vi "FPGA_PPG_stop.vi"(0 "resource_in":refnum<visa-resource-name>, 5 "error in (no error)":errorcluster) -> (14 "resource_out":refnum<visa-resource-name>, 16 "stop_addr":u32, 19 "error out":errorcluster)   [LabVIEW 2014, in "NI-FPGA_PPG_Driver.lvlib"]
doc: "Stops the FPGA and returns the last executed command specified by address.\n\nContact: Falk Ziegler, eMail: ziegler@physik.uni-greifswald.de"
uses:
  NI-FPGA_PPG_Driver.lvlib
  <vilib>/Utility/error.llb/Error Cluster From Error Code.vi
  <vilib>/rvi/errors/niLvFpgaAdjustHostInterfaceError.vi
  <vilib>/rvi/interface/nirviReadWriteControl/nirviReadWriteControl.xnode
  FPGA_PPG_vi_ref.ctl
  FPGA Bitfiles/TiTaProj_COF_PPG_d3vptxinz-s.lvbitx
  NiFpgaLv.dll
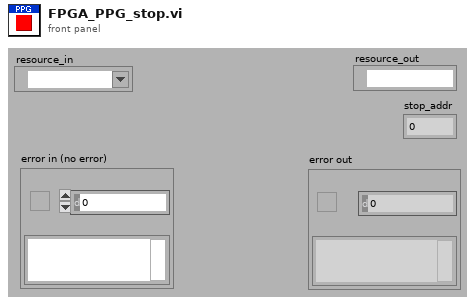
[diagram p1: front panel]
types:
  T1 = typedef "NI-FPGA_PPG_Driver.lvlib/FPGA_PPG_vi_ref.ctl" = refnum<k20>
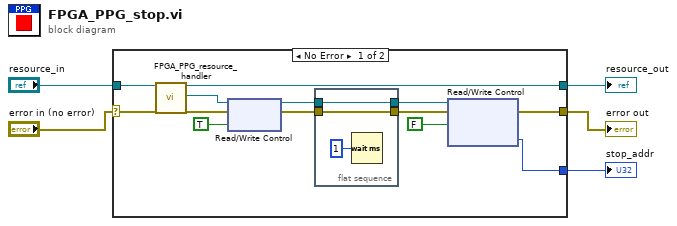
[diagram p0: block diagram]
diagram:
  n1 = case shown="No Error" "error in (no error)" {
    selector: "error in (no error)" -> [w17 w23]
    tunnel: [w8 w23] -> w4
    tunnel: "resource_in" -> [w18 w22]
    tunnel: [w7 w22] -> w2
    tunnel: [w9 _] -> w1
    frame No Error {
      n2 = call "FPGA_PPG_resource_handler.vi"("resource_in"=w18, "error in (no error)"=w17) -> ("resource_out"=w7:refnum<visa-resource-name>, "FPGA VI Reference Out"=w6:T1, "error out"=w16:errorcluster)  [unwired: 15 in]
      n3 = xnode "Read/Write Control"("FPGA VI Reference In"=w6, "error in"=w16, "stop"=TRUE) -> ("FPGA VI Reference Out"=w14:T1, "error out"=w13:errorcluster)
      n4 = flat-sequence {
        tunnel: w14 -> [w20]
        tunnel: w13 -> [w19]
        tunnel: [w20] -> w12
        tunnel: [w19] -> w11
        frame #0 {
          n5 = Wait (ms)(milliseconds to wait=u32 1) -> ()  [unwired: 1 out]
        }
      }
      n6 = xnode "Read/Write Control"("FPGA VI Reference In"=w12, "error in"=w11, "stop"=FALSE) -> ("error out"=w8:errorcluster, "stop_addr"=w9:u32)  [unwired: 1 out]
    }
    frame Error {
    }
  }
  "error out" <- w4
  "resource_out" <- w2
  "stop_addr" <- w1
